vi "Write Buttons_refs.vi"(8 "error in (no error)":errorcluster, 10 "input cluster":T1, 11 "Control-Server in":refnum<class "Control-Server.lvclass">) -> (0 "error out":errorcluster, 3 "Control-Server out":refnum<class "Control-Server.lvclass">)   [LabVIEW 2015, in "Control-Server.lvclass"]
uses:
  Control-Server.lvclass
  dependecies/ControlsVIs/Clusters-def/DEFs_SERVER_buttons_refs.ctl
  Control-Server.lvclass/Control-Server.ctl
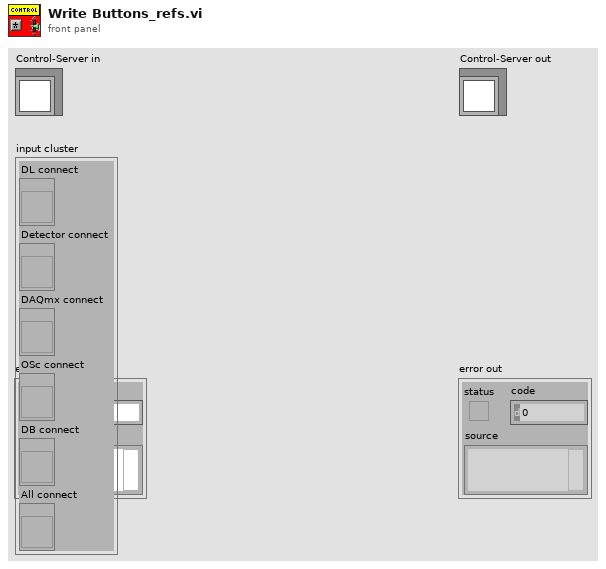
[diagram p1: front panel]
types:
  T1 = typedef "Control-Server.lvclass/DEFs_SERVER_buttons_refs.ctl" = cluster{"DL connect":refnum<vi>, "Detector connect":refnum<vi>, "DAQmx connect":refnum<vi>, "OSc connect":refnum<vi>, "DB connect":refnum<vi>, "All connect":refnum<vi>}
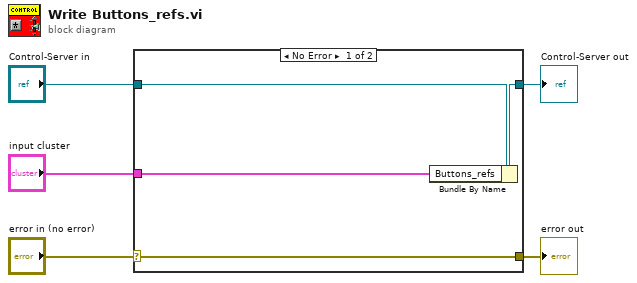
[diagram p0: block diagram]
diagram:
  n1 = case shown="No Error" "error in (no error)" {
    selector: "error in (no error)" -> [w9 w10]
    tunnel: [w9 w10] -> w4
    tunnel: [w7 w11] -> w2
    tunnel: "Control-Server in" -> [w8 w11]
    tunnel: "input cluster" -> [w6 _]
    frame No Error {
      n2 = Bundle By Name(cluster=w8, "Buttons_refs"=w6) -> (w7:refnum<class "Control-Server.lvclass">)
    }
    frame Error {
    }
  }
  "error out" <- w4
  "Control-Server out" <- w2
